vi "svx_Polar_Cursor_Info.vi"(4 "format string":string="%.1p", 6 "cursor color(blue)":u32(colorbox)=16860, 7 "Empty?":bool, 8 "mark unit":string, 9 "magnitude unit":string, 10 "CursLoc":T1, 11 "Polar Plot":refnum<vi>) -> (3 "cursor name":string)   [LabVIEW 2017, in "SVX Polar Plot.xctl"]
uses:
  <vilib>/addons/_XControls/Polar Plot/SVX Polar Plot.xctl
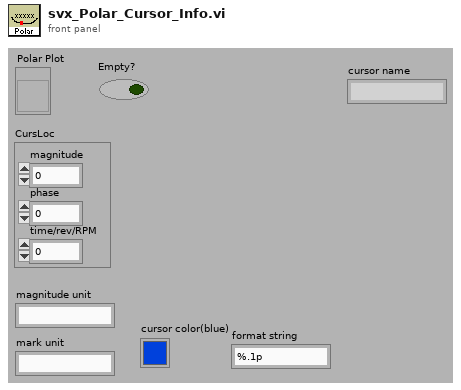
[diagram p1: front panel]
types:
  T1 = cluster{"magnitude":dbl, "phase":dbl, "time/rev/RPM":dbl}
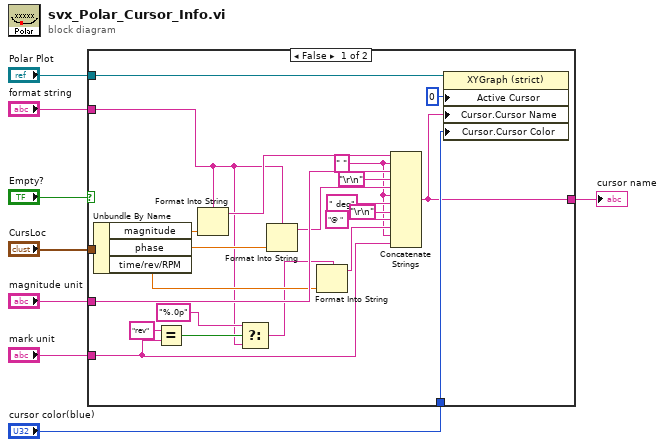
[diagram p0: block diagram]
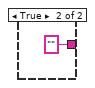
[diagram p2: hidden frame]
diagram:
  n1 = case shown="False" "Empty?" {
    tunnel: "cursor color(blue)" -> [w16 _]
    tunnel: "CursLoc" -> [w31 _]
    tunnel: "Polar Plot" -> [w18 _]
    tunnel: "format string" -> [w10 _]
    tunnel: "magnitude unit" -> [w27 _]
    tunnel: "mark unit" -> [w13 _]
    tunnel: [w15 ""] -> w2
    frame False {
      w19 = " " ("string")
      n2 = Unbundle By Name(w31) -> ("magnitude"=w29:dbl, "phase"=w28:dbl, "time/rev/RPM"=w23:dbl)
      n3 = Equal?(x="rev", y=w13) -> (x = y?=w12:bool)
      n4 = Format Into String(format string=w10, w29) -> (resulting string=w30:string)  [unwired: 2 in, 1 out]
      n5 = Select(t="%.0p" ("format string"), s=w12, f=w10) -> (s? t:f=w9:string)
      n6 = Format Into String(format string=w10, w28) -> (resulting string=w26:string)  [unwired: 2 in, 1 out]
      n7 = Format Into String(format string=w9, w23) -> (resulting string=w22:string)  [unwired: 2 in, 1 out]
      n8 = Concatenate Strings(w30, w19, w27, "\r\n", w26, w19, " deg" ("string"), "\r\n", "@ " ("string"), w22, w19, w13) -> (w15:string)
      n9 = property class="XYGraph (strict)"(reference=w18, "Active Cursor"=u32 0, "Cursor.Cursor Name"=w15, "Cursor.Cursor Color"=w16) -> ()  [unwired: 1 in, 2 out]
    }
    frame True {
    }
  }
  "cursor name" <- w2
